vi "Get Joystick Inputs.vi"(11 "Joystick Refnum":string="My Joystick RefNum") -> (3 "Joystick Output":T1)   [LabVIEW 2017]
uses:
  Controls/Joystick Controls.ctl
  <vilib>/Rock Robotics/WPI/Utilities/WPI_GetSetVariantRefNum.vi
panel:
  in  "Robot Controls":T1
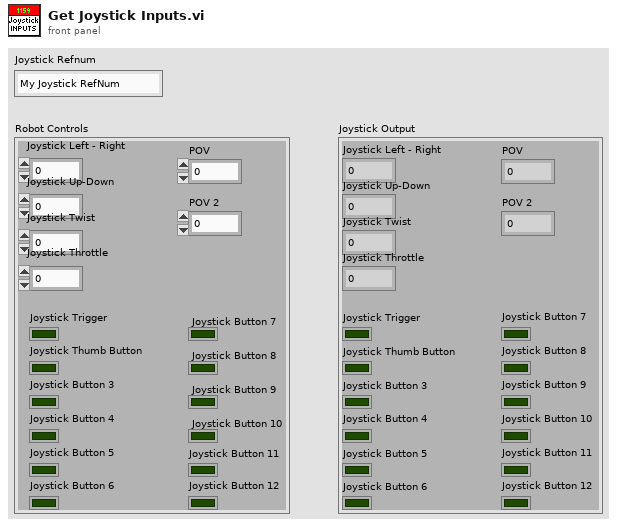
[diagram p1: front panel]
types:
  T1 = typedef "Joystick Controls.ctl" = cluster{"Joystick Left - Right":dbl, "Joystick Up-Down":dbl, "Joystick Twist":dbl, "Joystick Throttle":dbl, "Joystick Trigger":bool, "Joystick Thumb Button":bool, "Joystick Button 3":bool, "Joystick Button 4":bool, "Joystick Button 5":bool, "Joystick Button 6":bool, "Joystick Button 7":bool, "Joystick Button 8":bool, "Joystick Button 9":bool, "Joystick Button 10":bool, "Joystick Button 11":bool, "Joystick Button 12":bool, "POV":i16, "POV 2":i16}
  T2 = typedef "WPI_JoystickDevRef.ctl" = cluster{"Device":T3}
  T3 = typedef "WPI_JoystickDeviceEnum.ctl" = enum16{"USB 0", "USB 1", "USB 2", "USB 3", "USB 4", "USB 5"}
  T4 = cluster{"Axes[0]":dbl, "Axes[1]":dbl, "Axes[2]":dbl, "Axes[3]":dbl, "Axes[4]":dbl, "Axes[5]":dbl, "Axes[6]":dbl, "Axes[7]":dbl, "Axes[8]":dbl}
  T5 = cluster{"POVs[0]":i16, "POVs[1]":i16, "POVs[2]":i16, "POVs[3]":i16, "POVs[4]":i16, "POVs[5]":i16, "POVs[6]":i16, "POVs[7]":i16, "POVs[8]":i16}
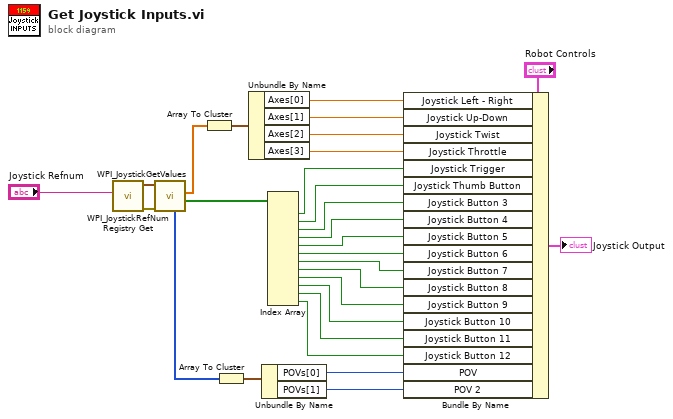
[diagram p0: block diagram]
diagram:
  n1 = call <vilib>:"WPI_JoystickRefNum Registry Get.vi"("refnum name"="Joystick Refnum") -> ("error out"=w3:errorcluster, "JoystickDevRef"=w28:T2)  [unwired: 9 in]
  n2 = call <vilib>:"WPI_JoystickGetValues.vi"("error in (no error)"=w3, "JoystickDevRef"=w28) -> ("Buttons"=w25:bool[], "Axes"=w26:dbl[], "POVs"=w16:i16[])  [unwired: 5 in, 2 out]
  n3 = Array To Cluster(array=w26) -> (cluster=w24:T4)
  n4 = Array To Cluster(array=w16) -> (cluster=w15:T5)
  n5 = Unbundle By Name(w24) -> ("Axes[0]"=w23:dbl, "Axes[1]"=w22:dbl, "Axes[2]"=w21:dbl, "Axes[3]"=w20:dbl)
  n6 = Unbundle By Name(w15) -> ("POVs[0]"=w14:i16, "POVs[1]"=w13:i16)
  n7 = Index Array(array=w25) -> (element #1=w19:bool, element #2=w18:bool, element #3=w17:bool, element #4=w12:bool, element #5=w11:bool, element #6=w10:bool, element #7=w9:bool, element #8=w8:bool, element #9=w7:bool, element #10=w6:bool, element #11=w5:bool, element #12=w4:bool)  [unwired: 12 in]
  n8 = Bundle By Name(cluster="Robot Controls", "Joystick Left - Right"=w23, "Joystick Up-Down"=w22, "Joystick Twist"=w21, "Joystick Throttle"=w20, "Joystick Trigger"=w19, "Joystick Thumb Button"=w18, "Joystick Button 3"=w17, "Joystick Button 4"=w12, "Joystick Button 5"=w11, "Joystick Button 6"=w10, "Joystick Button 7"=w9, "Joystick Button 8"=w8, "Joystick Button 9"=w7, "Joystick Button 10"=w6, "Joystick Button 11"=w5, "Joystick Button 12"=w4, "POV"=w14, "POV 2"=w13) -> (→"Joystick Output":T1)
